vi "heart rate NEW.vi"() -> ()   [LabVIEW 2019]
uses:
  <vilib>/httpClient/LabVIEWHTTPClient.lvlib
panel:
  in  "String":string
  out "NORMAL":bool
  in  "stop":bool
  out "TACHYCARDIA":bool
  out "BRADYCARDIA":bool
  out "CRUDE HEART RATE MONITOR":dbl(slide) scale=0.0..150.0
  in  "CRUDE HEART MONITOR":dbl(slide) scale=0.0..150.0
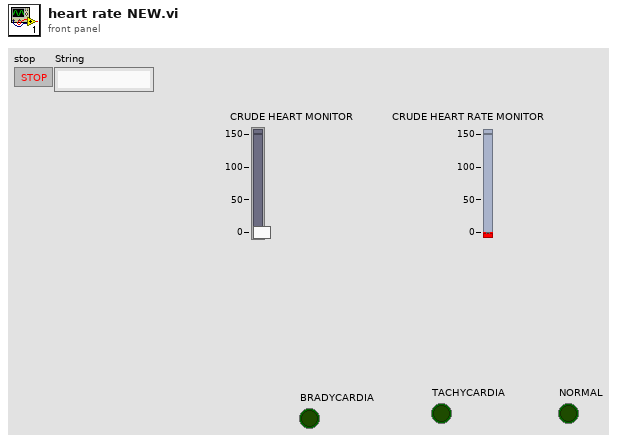
[diagram p1: front panel]
types:
  T1 = typedef "LabVIEWHTTPClient.lvlib/ClientHandle.ctl" = refnum<k1>
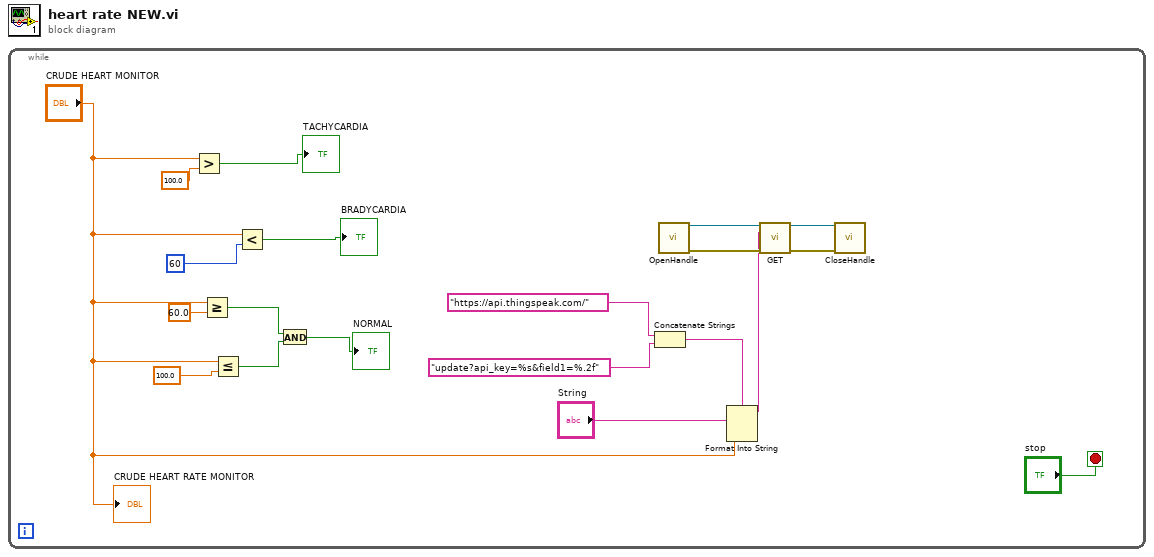
[diagram p0: block diagram]
diagram:
  n1 = while {
    stop <- "stop" stop-if-true
    n2 = Greater?(x="CRUDE HEART MONITOR", y=100.0 ("x")) -> (0:→"TACHYCARDIA":bool)
    n3 = Greater Or Equal?(x="CRUDE HEART MONITOR", y=60.0) -> (x >= y?=w17:bool)
    n4 = Less Or Equal?(x="CRUDE HEART MONITOR", y=100.0 ("x")) -> (x <= y?=w16:bool)
    n5 = Less?(x="CRUDE HEART MONITOR", y=u64 60 ("x")) -> (x < y?=→"BRADYCARDIA":bool)
    n6 = And(x=w17, y=w16) -> (x .and. y?=→"NORMAL":bool)
    n7 = Concatenate Strings("https://api.thingspeak.com/", "update?api_key=%s&field1=%.2f") -> (w4:string)
    n8 = call <vilib>:"OpenHandle.vi"() -> ("client handle out"=w12:T1, "error out"=w11:errorcluster)  [unwired: 14 in]
    n9 = Format Into String(format string=w4, "String", "CRUDE HEART MONITOR") -> (resulting string=w1:string)  [unwired: 2 in, 1 out]
    n10 = call <vilib>:"GET.vi"("client handle"=w12, "url"=w1, "error in (no error)"=w11) -> ("client handle out"=w9:T1, "error out"=w10:errorcluster)  [unwired: 9 in, 2 out]
    n11 = call <vilib>:"CloseHandle.vi"("client handle"=w9, "error in (no error)"=w10) -> ()  [unwired: 13 in, 1 out]
    "CRUDE HEART RATE MONITOR" <- "CRUDE HEART MONITOR"
  }
